vi "spect_test_init.vi"(8 "error in":errorcluster, 10 "buffer size (in samples per channel)":u32=500000, 11 "Configuration in":T1) -> (0 "error out":errorcluster, 3 "Configuration out":T1)   [LabVIEW 2012]
uses:
  initialization/configuration.ctl
  initialization/asap_calibration.ctl
  <vilib>/Analysis/Matrix/Datatypes/RealMatrix.ctl
  <vilib>/DAQmx/create/channels.llb/DAQmx Create Channel (AI-Voltage-Basic).vi
  initialization/globals.vi
  <vilib>/DAQmx/configure/timing.llb/DAQmx Timing (Sample Clock).vi
  <vilib>/Analysis/Matrix/NI_Matrix.lvlib
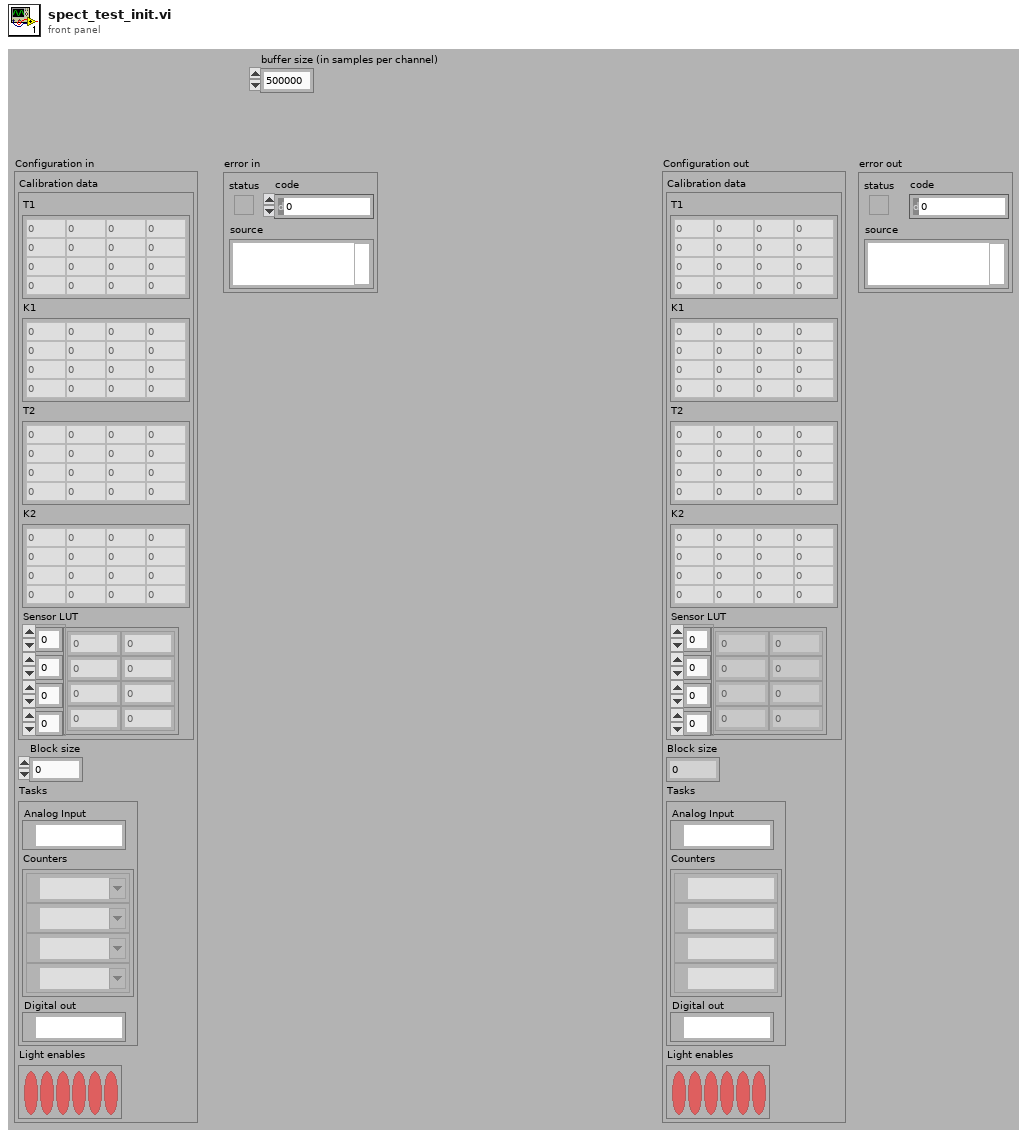
[diagram p1: front panel]
types:
  T1 = typedef "configuration.ctl" = cluster{"Calibration data":T2, "Block size":i32, "Tasks":cluster{"Analog Input":refnum<k21>, "Counters":refnum<k21>[], "Digital out":refnum<k21>}, "Light enables":bool[]}
  T2 = typedef "asap_calibration.ctl" = cluster{"T1":T3, "K1":T3, "T2":T3, "K2":T3, "Sensor LUT":sgl[][][][]}
  T3 = typedef "NI_Matrix.lvlib/RealMatrix.ctl" = dbl[][]
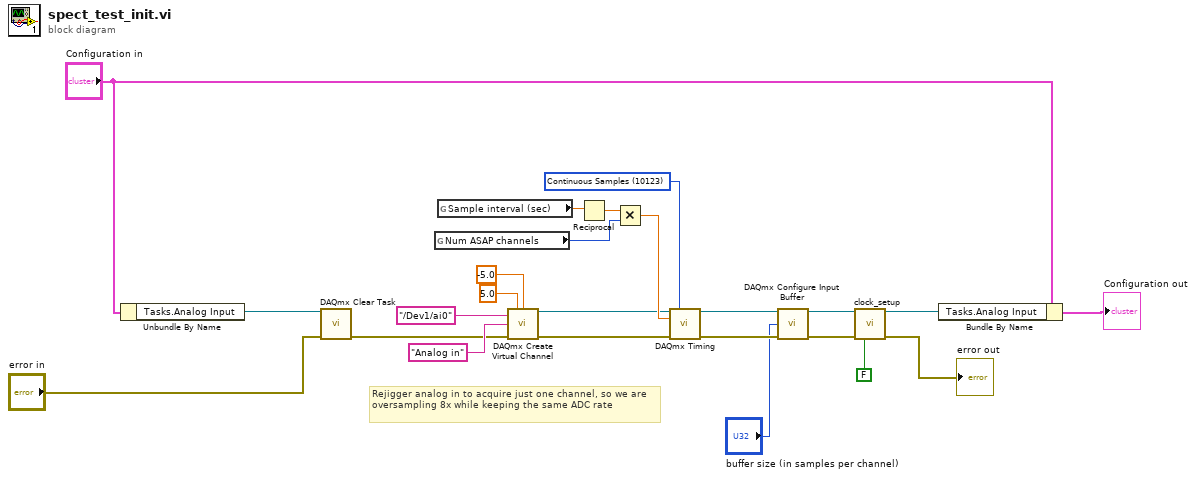
[diagram p0: block diagram]
diagram:
  w19 = 10123 items=["Finite Samples"=10178, "Continuous Samples"=10123, "Hardware Timed Single Point"=12522] ("sample mode")
  # "Rejigger analog in to acquire just one channel, so we are oversampling 8x while keeping the same ADC rate"
  n1 = Unbundle By Name("Configuration in") -> ("Tasks.Analog Input"=w17:refnum<k21>)
  n2 = call <vilib>:"DAQmx Clear Task.vi"("task in"=w17, "error in"="error in") -> ("error out"=w11:errorcluster)  [unwired: 13 out]
  n3 = global read "globals.vi" "Num ASAP channels"() -> (w21:i32)
  n4 = global read "globals.vi" "Sample interval (sec)"() -> (w18:dbl)
  n5 = call-poly <vilib>:"DAQmx Create Virtual Channel.vi"("maximum value"=5.0, "minimum value"=-5.0 ("maximum value"), "physical channels"="/Dev1/ai0", "name to assign"="Analog in", "error in"=w11) -> ("task out"=w9:refnum<k21>, "error out"=w8:errorcluster)  [unwired: 4 in, 5 out]
  n6 = Reciprocal(x=w18) -> (1/x=w20:dbl)
  n7 = Multiply(x=w20, y=w21) -> (x*y=w24:dbl)
  n8 = call-poly <vilib>:"DAQmx Timing.vi"("task/channels in"=w9, "sample mode"=w19, "rate"=w24, "error in"=w8) -> ("task out"=w5:refnum<k21>, "error out"=w4:errorcluster)  [unwired: 3 in, 7 out]
  n9 = call <vilib>:"DAQmx Configure Input Buffer.vi"("task/channels in"=w5, "buffer size (in samples per channel)"="buffer size (in samples per channel)", "error in"=w4) -> ("task out"=w2:refnum<k21>, "error out"=w3:errorcluster)  [unwired: 11 in]
  n10 = call "clock_setup.vi"("task in"=w2, "error in"=w3, "Dev2"=FALSE) -> ("task out"=w6:refnum<k21>, "error out"=→"error out":errorcluster)  [unwired: 11 in]
  n11 = Bundle By Name(cluster="Configuration in", "Tasks.Analog Input"=w6) -> (→"Configuration out":T1)
